vi "Reentrant.vi"() -> (1 "NumOut":dbl)   [LabVIEW 2012]
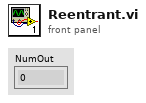
[diagram p1: front panel]
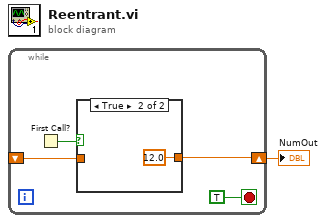
[diagram p0: block diagram]
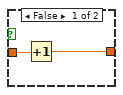
[diagram p2: hidden frame]
diagram:
  n1 = while {
    shift-right: [w5] -> w1
    shift-left: _ -> [w4]
    stop <- TRUE stop-if-true
    n2 = First Call?() -> (First Call?: T/F=w2:bool)
    n3 = case shown="True" w2 {
      tunnel: [w7 12.0] -> w5
      tunnel: w4 -> [w6 _]
      frame False {
        n4 = Increment(x=w6) -> (x+1=w7:dbl)
      }
      frame True {
      }
    }
  }
  "NumOut" <- w1
